vi "Lambdaberechnung.vi"(9 "Nenner":u16, 10 "LowByte":u8, 11 "HighByte":u8) -> (1 "Wert":sgl)   [LabVIEW 2020, in "Lambda_ Komm.lvlib"]
uses:
  Lambda_ Komm.lvlib
panel:
  # "Lambda: 1000\nRi:           10\nA/F, O2:  100"
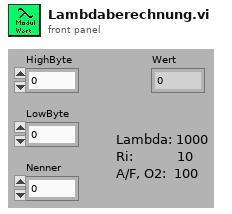
[diagram p1: front panel]
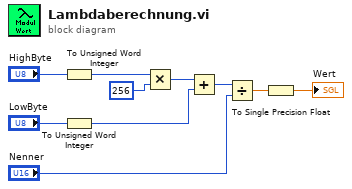
[diagram p0: block diagram]
diagram:
  n1 = To Unsigned Word Integer(number="HighByte") -> (unsigned 16bit integer=w5:u16)
  n2 = To Unsigned Word Integer(number="LowByte") -> (unsigned 16bit integer=w3:u16)
  n3 = Multiply(x=w5, y=u16 256) -> (x*y=w10:u16)
  n4 = Add(x=w10, y=w3) -> (x+y=w9:u16)
  n5 = Divide(x=w9, y="Nenner") -> (x/y=w2:dbl)
  n6 = To Single Precision Float(number=w2) -> (single precision float=→"Wert":sgl)
